vi "Set_360LED_power.vi"() -> ()   [LabVIEW 2014]
panel:
  in  "stop":bool
  in  "Power (0 - 5V)":dbl
  in  "Slide":dbl(slide) scale=0.0..5.0
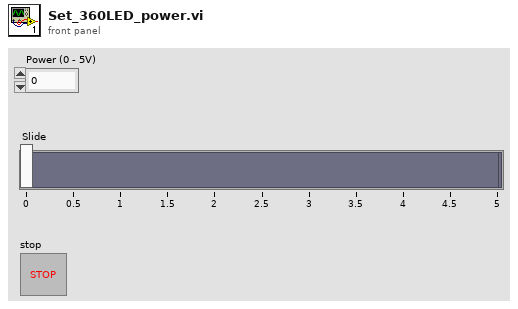
[diagram p1: front panel]
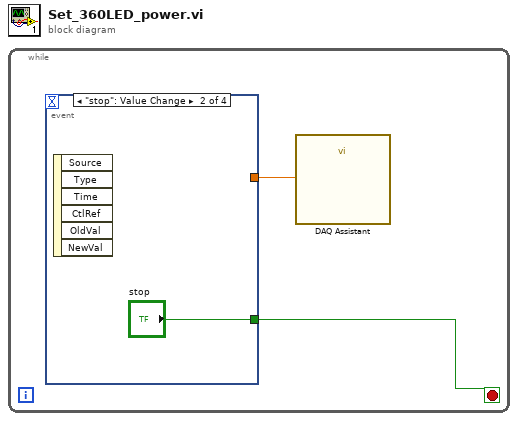
[diagram p0: block diagram]
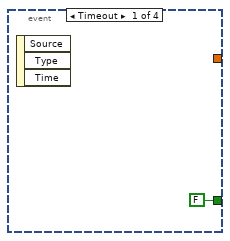
[diagram p2: hidden frame]
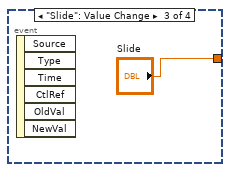
[diagram p3: hidden frame]
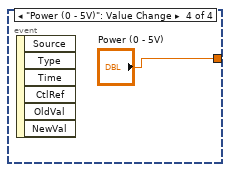
[diagram p4: hidden frame]
diagram:
  n1 = while {
    stop <- w1 stop-if-true
    n2 = event shown="[1] \"stop\": Value Change" {
      selector: _ -> [_ _ _ _]
      dyn-events: _ -> [_ _ _ _]
      timeout: _ -> [_ _ _ _]
      tunnel: [_ _ "Slide" "Power (0 - 5V)"] -> w2
      tunnel: [FALSE ("stop") "stop" _ _] -> w1
      event Timeout {
        n3 = event-data() -> ()  [unwired: 1 in, 3 out]
      }
      event "stop": Value Change {
        n4 = event-data() -> ()  [unwired: 1 in, 6 out]
      }
      event "Slide": Value Change {
        n5 = event-data() -> ()  [unwired: 1 in, 6 out]
      }
      event "Power (0 - 5V)": Value Change {
        n6 = event-data() -> ()  [unwired: 1 in, 6 out]
      }
    }
    n7 = call "DAQ Assistant"("data"=w2) -> ()  [unwired: 17 in, 2 out]
  }
